vi "Check Size Equality.vi"(7 "Command/Response Refnum in":T1 format="%.0x", 8 "Error In":errorcluster, 9 "Variables":string[](array[string]), 11 "Linked Channels in":cluster{"Variable Name":string, "GUID":string}[](array[cluster])) -> (0 "Error Out":errorcluster, 1 "Variables out":string[](array[string]), 3 "Linked Channels out":cluster{"Variable Name":string, "GUID":string}[](array[cluster]))   [LabVIEW 2018, in "Instrument Addon Scripting API.lvlib"]
uses:
  Instrument Addon Scripting API.lvlib
  <vilib>/NI Veristand/Custom Device API/Custom Device Item Ref.ctl
  Addon/Addon Shared/SubVIs/Constants.vi
  Addon/Addon Shared/Instrument Addon Shared.lvlib
  <vilib>/NI VeriStand/Custom Device API/Custom Device API.lvlib
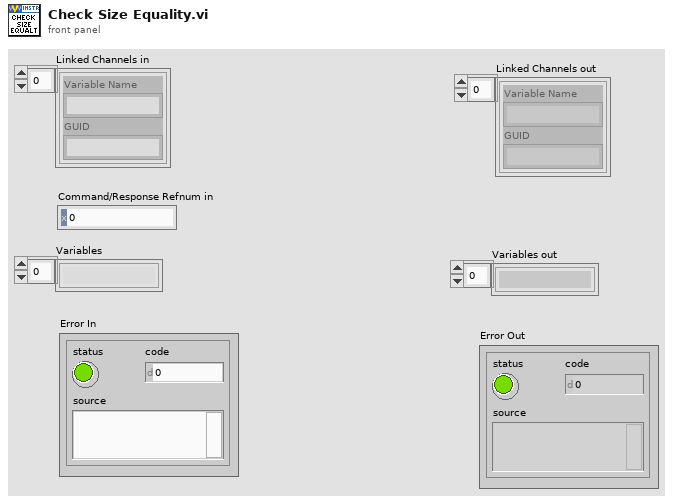
[diagram p1: front panel]
types:
  T1 = typedef "Custom Device API.lvlib/Custom Device Item Ref.ctl" = u64
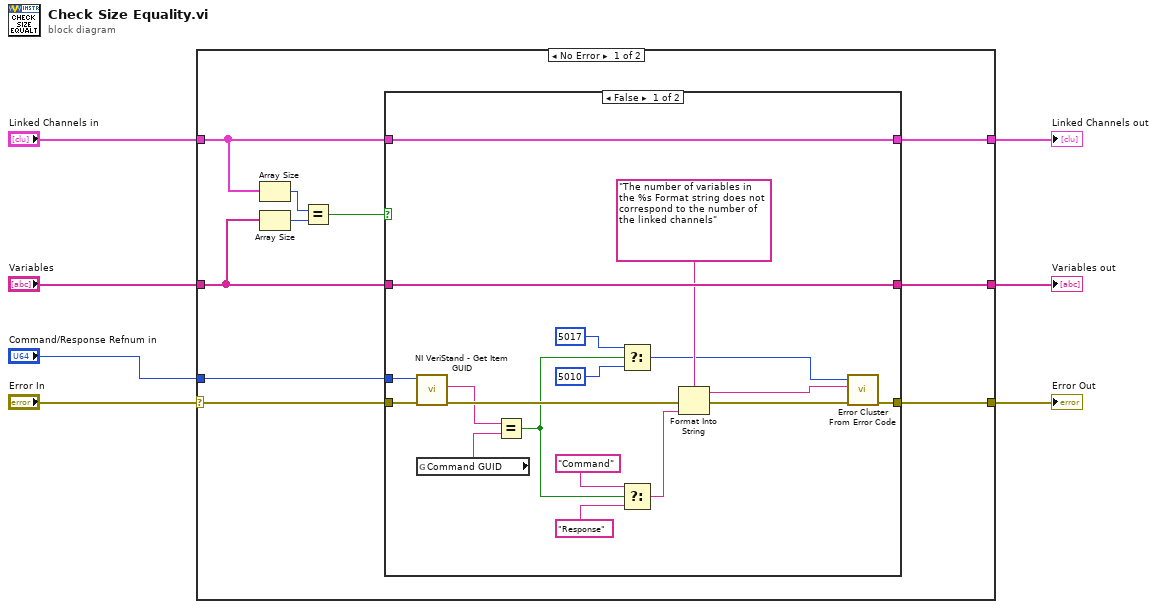
[diagram p0: block diagram]
diagram:
  n1 = case shown="No Error" "Error In" {
    selector: "Error In" -> [w14 w41]
    tunnel: "Variables" -> [w12 w39]
    tunnel: "Linked Channels in" -> [w11 w40]
    tunnel: [w13 w41] -> w4
    tunnel: [w10 w40] -> w3
    tunnel: [w9 w39] -> w2
    tunnel: "Command/Response Refnum in" -> [w8 _]
    frame No Error {
      n2 = Array Size(array=w11) -> (size(s)=w17:i32)
      n3 = Array Size(array=w12) -> (size(s)=w16:i32)
      n4 = Equal?(x=w17, y=w16) -> (x = y?=w15:bool)
      n5 = case shown="False" w15 {
        tunnel: w14 -> [w31 w38]
        tunnel: [w35 w38] -> w13
        tunnel: w12 -> [w33 w36]
        tunnel: w11 -> [w34 w37]
        tunnel: [w34 w37] -> w10
        tunnel: [w33 w36] -> w9
        tunnel: w8 -> [w32 _]
        frame False {
          n6 = call <vilib>:"NI VeriStand - Get Item GUID.vi"("error in (no error)"=w31, "Item Ref in"=w32) -> ("error out"=w26:errorcluster, "GUID"=w23:string)  [unwired: 7 in, 1 out]
          n7 = global read "Constants.vi" "Command GUID"() -> (w22:string)
          n8 = Equal?(x=w23, y=w22) -> (x = y?=w21:bool)
          n9 = Select(t=5017 ("error code (0)"), s=w21, f=5010 ("error code (0)")) -> (s? t:f=w18:i32)
          n10 = Select(t="Command", s=w21, f="Response") -> (s? t:f=w27:string)
          n11 = Format Into String(format string="The number of variables in the %s Format string does not correspond to the number of the linked channels" ("error message (\"\")"), error in=w26, w27) -> (resulting string=w24:string, error out=w25:errorcluster)  [unwired: 1 in]
          n12 = call <vilib>:"Error Cluster From Error Code.vi"("error in (no error)"=w25, "error message (\"\")"=w24, "error code (0)"=w18) -> ("error out"=w35:errorcluster)  [unwired: 6 in]
        }
        frame True {
        }
      }
    }
    frame Error {
    }
  }
  "Error Out" <- w4
  "Linked Channels out" <- w3
  "Variables out" <- w2
